vi "Multiple Connections - Server - TCP - 複製.vi"() -> ()   [LabVIEW 2011]
doc: "Demonstrates how to establish multiple connections and place them in a queue to be serviced. As connections are made, it sends the current date and time via TCP to all Client VIs that connect to it.\n\nThis VI has two parts -- a loop that listens for each client to connect, and a loop that sends the date and time to each connection in the queue.\n\n<B>Note:</B> Use this VI with Multiple Connections - Client 1.vi and Multiple Connections - Client 2.vi."
panel:
  out "# 2":i32
  in  "Port 2":u16=6342
  in  "stop":bool=TRUE
  out "# of Connections":i32
  in  "Port":u16=6341
  # "TCP Information"
  # "Instructions:\n1. Open the Multiple Connections - Client 1 and Client 2 VIs.\n2. Run this VI first.\n3. Run the Client VIs second and follow the instructions on their front panels.\n4. Stop This VI.  The Client VIs will stop on their own when they time out."
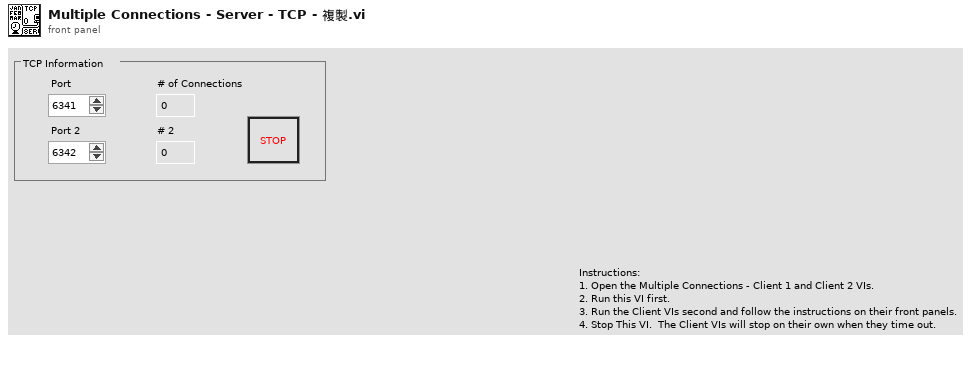
[diagram p1: front panel]
types:
  T1 = enum16{"Obtain", "Enqueue", "Dequeue", "Release"}
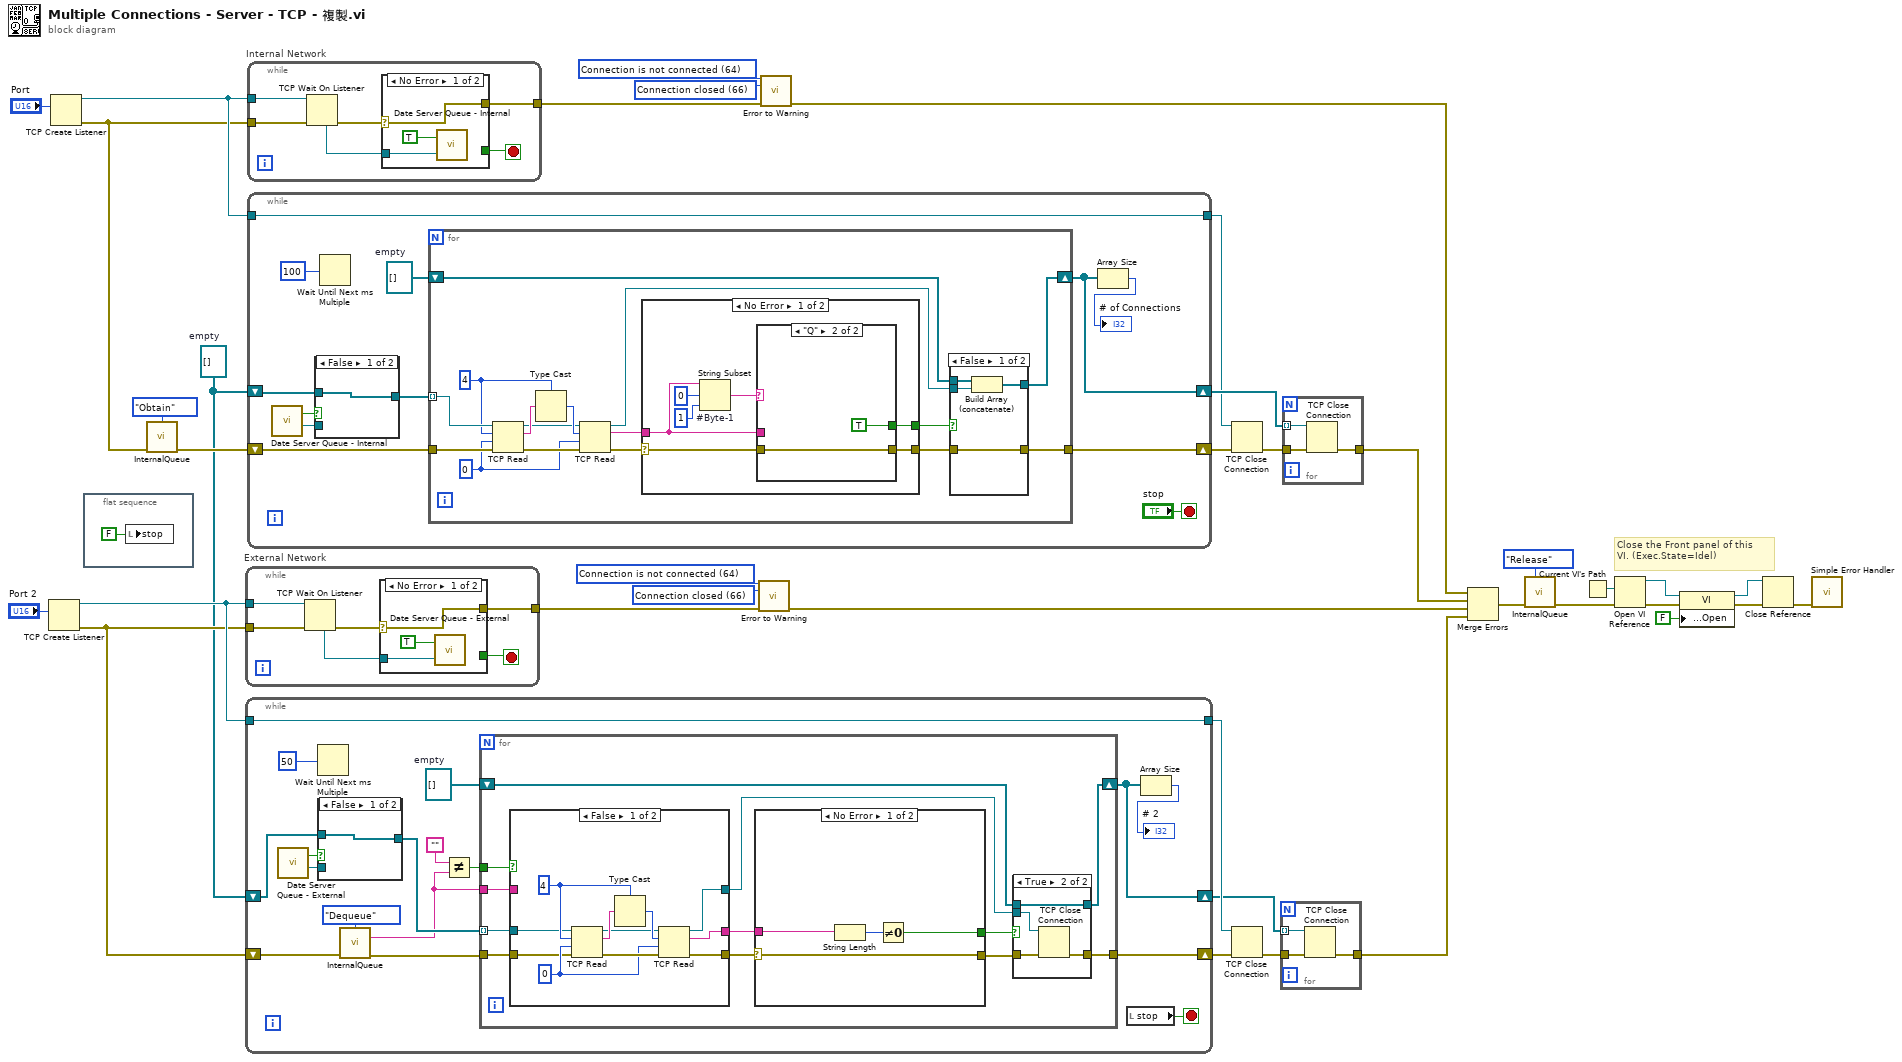
[diagram p0: block diagram]
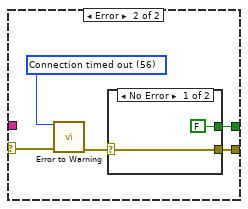
[diagram p2: hidden frame]
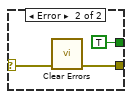
[diagram p3: hidden frame]
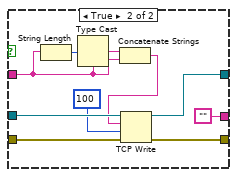
[diagram p4: hidden frame]
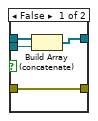
[diagram p5: hidden frame]
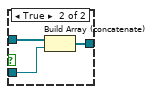
[diagram p6: hidden frame]
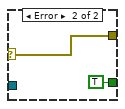
[diagram p7: hidden frame]
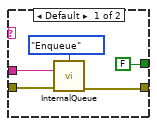
[diagram p8: hidden frame]
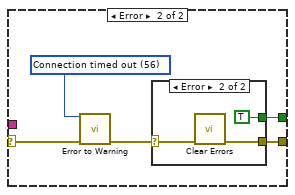
[diagram p9: hidden frame]
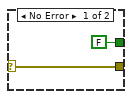
[diagram p10: hidden frame]
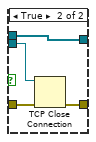
[diagram p11: hidden frame]
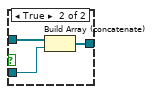
[diagram p12: hidden frame]
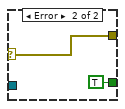
[diagram p13: hidden frame]
diagram:
  w20 = 66 items=["No Error", "Argument Error", "Memory Full", "Out of Zone", "End of File", "File Already Open", "Generic File IO Error", "File Not Found", "File Permission Error", "Disk Full", "Duplicate Path", "Too Many Files Open", "Not Enabled", "Resource File Not Found", "Cannot Add Resource", "Resource Not Found", "Image Not Found", "Image Memory Error", "Pen Does Not Exist", "Config Bad Type", "Config Token Not Found", "Config Parse Error", "Config Memory Error", "Bad External Code Format", "Bad External Code Offset", "External Code Not Present", "Null Window", "Destroy Window Mixup", "Null Menu", "Print Aborted", "Bad Print Record", "Print Driver Error", "Windows Error During Print", "Memory Error During Print", "Print Dialog Error", "Generic Print Error", "Invalid Device Refnum", "Device Not Found", "Device Parameter Error", "Device Unit Error", "Can't Open Device", "Device Call Aborted", "Generic Error", "Cancelled By User", "Object ID Too Low", "Object ID Too High", "Object Not In Heap", "Unknown Heap", "Bad DefProc ID", "DefProc Not In Table", "Message Out Of Range", "Null Method", "Unknown Message", "Manager Call Not Supported", "Bad address", "Connection In progress", "Connection timed out", "Connection is already in progress", "Network attribute not supported", "Network error", "Address in use", "System out of memory", "Connection aborted", "Connection refused", "Connection is not connected", "Connection is already connected", "Connection closed", "Initialize error (interapplication manager)", "Bad occurrence", "Wait on unbound occurrence handler", "Occurrence queue overflow", "Bad path", "Semaphore not signaled", "Unrecognized type (interapplication manager)"] ("2nd Error to Convert")
  w19 = 64 items=["No Error", "Argument Error", "Memory Full", "Out of Zone", "End of File", "File Already Open", "Generic File IO Error", "File Not Found", "File Permission Error", "Disk Full", "Duplicate Path", "Too Many Files Open", "Not Enabled", "Resource File Not Found", "Cannot Add Resource", "Resource Not Found", "Image Not Found", "Image Memory Error", "Pen Does Not Exist", "Config Bad Type", "Config Token Not Found", "Config Parse Error", "Config Memory Error", "Bad External Code Format", "Bad External Code Offset", "External Code Not Present", "Null Window", "Destroy Window Mixup", "Null Menu", "Print Aborted", "Bad Print Record", "Print Driver Error", "Windows Error During Print", "Memory Error During Print", "Print Dialog Error", "Generic Print Error", "Invalid Device Refnum", "Device Not Found", "Device Parameter Error", "Device Unit Error", "Can't Open Device", "Device Call Aborted", "Generic Error", "Cancelled By User", "Object ID Too Low", "Object ID Too High", "Object Not In Heap", "Unknown Heap", "Bad DefProc ID", "DefProc Not In Table", "Message Out Of Range", "Null Method", "Unknown Message", "Manager Call Not Supported", "Bad address", "Connection In progress", "Connection timed out", "Connection is already in progress", "Network attribute not supported", "Network error", "Address in use", "System out of memory", "Connection aborted", "Connection refused", "Connection is not connected", "Connection is already connected", "Connection closed", "Initialize error (interapplication manager)", "Bad occurrence", "Wait on unbound occurrence handler", "Occurrence queue overflow", "Bad path", "Semaphore not signaled", "Unrecognized type (interapplication manager)"] ("1st Error to Convert")
  w11 = refnum<k5>[] []  # empty
  w32 = 66 items=["No Error", "Argument Error", "Memory Full", "Out of Zone", "End of File", "File Already Open", "Generic File IO Error", "File Not Found", "File Permission Error", "Disk Full", "Duplicate Path", "Too Many Files Open", "Not Enabled", "Resource File Not Found", "Cannot Add Resource", "Resource Not Found", "Image Not Found", "Image Memory Error", "Pen Does Not Exist", "Config Bad Type", "Config Token Not Found", "Config Parse Error", "Config Memory Error", "Bad External Code Format", "Bad External Code Offset", "External Code Not Present", "Null Window", "Destroy Window Mixup", "Null Menu", "Print Aborted", "Bad Print Record", "Print Driver Error", "Windows Error During Print", "Memory Error During Print", "Print Dialog Error", "Generic Print Error", "Invalid Device Refnum", "Device Not Found", "Device Parameter Error", "Device Unit Error", "Can't Open Device", "Device Call Aborted", "Generic Error", "Cancelled By User", "Object ID Too Low", "Object ID Too High", "Object Not In Heap", "Unknown Heap", "Bad DefProc ID", "DefProc Not In Table", "Message Out Of Range", "Null Method", "Unknown Message", "Manager Call Not Supported", "Bad address", "Connection In progress", "Connection timed out", "Connection is already in progress", "Network attribute not supported", "Network error", "Address in use", "System out of memory", "Connection aborted", "Connection refused", "Connection is not connected", "Connection is already connected", "Connection closed", "Initialize error (interapplication manager)", "Bad occurrence", "Wait on unbound occurrence handler", "Occurrence queue overflow", "Bad path", "Semaphore not signaled", "Unrecognized type (interapplication manager)"] ("2nd Error to Convert")
  w33 = 64 items=["No Error", "Argument Error", "Memory Full", "Out of Zone", "End of File", "File Already Open", "Generic File IO Error", "File Not Found", "File Permission Error", "Disk Full", "Duplicate Path", "Too Many Files Open", "Not Enabled", "Resource File Not Found", "Cannot Add Resource", "Resource Not Found", "Image Not Found", "Image Memory Error", "Pen Does Not Exist", "Config Bad Type", "Config Token Not Found", "Config Parse Error", "Config Memory Error", "Bad External Code Format", "Bad External Code Offset", "External Code Not Present", "Null Window", "Destroy Window Mixup", "Null Menu", "Print Aborted", "Bad Print Record", "Print Driver Error", "Windows Error During Print", "Memory Error During Print", "Print Dialog Error", "Generic Print Error", "Invalid Device Refnum", "Device Not Found", "Device Parameter Error", "Device Unit Error", "Can't Open Device", "Device Call Aborted", "Generic Error", "Cancelled By User", "Object ID Too Low", "Object ID Too High", "Object Not In Heap", "Unknown Heap", "Bad DefProc ID", "DefProc Not In Table", "Message Out Of Range", "Null Method", "Unknown Message", "Manager Call Not Supported", "Bad address", "Connection In progress", "Connection timed out", "Connection is already in progress", "Network attribute not supported", "Network error", "Address in use", "System out of memory", "Connection aborted", "Connection refused", "Connection is not connected", "Connection is already connected", "Connection closed", "Initialize error (interapplication manager)", "Bad occurrence", "Wait on unbound occurrence handler", "Occurrence queue overflow", "Bad path", "Semaphore not signaled", "Unrecognized type (interapplication manager)"] ("1st Error to Convert")
  # "Close the Front panel of this\nVI. (Exec.State=Idel)"
  n1 = TCP Create Listener(10:"Port 2") -> (0:w12:errorcluster, 3:w17:refnum<k5>)  [unwired: 1 in, 4 out]
  n2 = TCP Create Listener(10:"Port") -> (0:w26:errorcluster, 3:w35:refnum<k5>)  [unwired: 1 in, 4 out]
  n3 = flat-sequence {
    frame #0 {
      n4 = local write "stop"(FALSE ("stop")) -> ()
    }
  }
  n5 = call "InternalQueue.vi"("Mode"=T1."Obtain", "error in (no error)"=w26) -> ("error out"=w28:errorcluster)  [unwired: 12 in, 1 out]
  n6 = while "External Network" {
    tunnel: w17 -> [w43]
    tunnel: w12 -> [w44]
    tunnel: [w39] -> w18
    stop <- w40 stop-if-true
    n7 = TCP Wait On Listener(8:w44, 11:w43) -> (0:w41:errorcluster, 4:w42:refnum<k5>)  [unwired: 5 out]
    n8 = case shown="No Error" w41 {
      selector: w41 -> [w45 w48]
      tunnel: w42 -> [w46 _]
      tunnel: [_ TRUE] -> w40
      tunnel: [w45 w48] -> w39
      frame No Error {
        n9 = call "Date Server Queue - External.vi"("new value"=w46, "set queue? (F: de-queue)"=TRUE) -> ()  [unwired: 2 out]
      }
      frame Error {
      }
    }
  }
  n10 = while {
    shift-left: w11 -> [w64]
    shift-right: [w61] -> w15
    tunnel: w17 -> [w59]
    tunnel: [w59] -> w16
    shift-right: [w58] -> w23
    shift-left: w12 -> [w56]
    stop <- w54 stop-if-true
    w62 = refnum<k5>[] []  # empty
    n11 = call "Date Server Queue - External.vi"() -> ("value"=w66:refnum<k5>, "valid?"=w65:bool)  [unwired: 2 in]
    n12 = Wait Until Next ms Multiple(millisecond multiple=u32 50) -> ()  [unwired: 1 out]
    n13 = case shown="False" w65 {
      tunnel: w66 -> [_ w125]
      tunnel: w64 -> [w122 w124]
      tunnel: [w122 w123] -> w63
      frame False {
      }
      frame True {
        n14 = Build Array (concatenate)(w124, w125) -> (w123:refnum<k5>[])
      }
    }
    n15 = call "InternalQueue.vi"("Mode"=T1."Dequeue", "error in (no error)"=w56) -> ("Queue Out"=w51:string, "error out"=w55:errorcluster)  [unwired: 12 in]
    n16 = Not Equal?(x="", y=w51) -> (x != y?=w50:bool)
    n17 = for {
      tunnel: w63 -> [w75] mode=indexing
      shift-right: [w76] -> w61
      shift-left: w62 -> [w78]
      tunnel: [w77] -> w58
      tunnel: w55 -> [w74]
      tunnel: w51 -> [w69]
      tunnel: w50 -> [w68]
      n18 = case shown="False" w68 {
        tunnel: w75 -> [w95 w109]
        tunnel: w74 -> [w97 w111]
        tunnel: [w96 w107] -> w73
        tunnel: w69 -> [_ w110]
        tunnel: [w93 w105] -> w67
        tunnel: [w94 ""] -> w70
        frame False {
          w98 = 0 ("timeout ms (25000)")
          w100 = 4
          n19 = TCP Read(connection ID=w95, bytes to read=w100, error in (no error)=w97, 9:w98) -> (connection ID out=w99:refnum<k5>, data out=w101:string, error out=w102:errorcluster)  [unwired: 1 out]
          n20 = Type Cast(type=w100, x=w101) -> (*(type *) &x=w103:i32)
          n21 = TCP Read(connection ID=w99, bytes to read=w103, error in (no error)=w102, 9:w98) -> (connection ID out=w93:refnum<k5>, data out=w94:string, error out=w96:errorcluster)  [unwired: 1 out]
        }
        frame True {
          n22 = String Length(string=w110) -> (length=w113:i32)
          n23 = Type Cast(type=w110, x=w113) -> (*(type *) &x=w112:string)
          n24 = Concatenate Strings(w112, w110) -> (w106:string)
          n25 = TCP Write(connection ID=w109, data in=w106, error in (no error)=w111, 9:100 ("timeout ms (25000)")) -> (connection ID out=w105:refnum<k5>, error out=w107:errorcluster)  [unwired: 1 out]
        }
      }
      n26 = case shown="No Error" w73 {
        selector: w73 -> [w82 w87]
        tunnel: [w82 w84] -> w71
        tunnel: [w79 w83] -> w72
        tunnel: w70 -> [w81 _]
        frame No Error {
          n27 = String Length(string=w81) -> (length=w80:i32)
          n28 = Not Equal To 0?(x=w80) -> (x != 0?=w79:bool)
        }
        frame Error {
          w86 = 56 items=["No Error", "Argument Error", "Memory Full", "Out of Zone", "End of File", "File Already Open", "Generic File IO Error", "File Not Found", "File Permission Error", "Disk Full", "Duplicate Path", "Too Many Files Open", "Not Enabled", "Resource File Not Found", "Cannot Add Resource", "Resource Not Found", "Image Not Found", "Image Memory Error", "Pen Does Not Exist", "Config Bad Type", "Config Token Not Found", "Config Parse Error", "Config Memory Error", "Bad External Code Format", "Bad External Code Offset", "External Code Not Present", "Null Window", "Destroy Window Mixup", "Null Menu", "Print Aborted", "Bad Print Record", "Print Driver Error", "Windows Error During Print", "Memory Error During Print", "Print Dialog Error", "Generic Print Error", "Invalid Device Refnum", "Device Not Found", "Device Parameter Error", "Device Unit Error", "Can't Open Device", "Device Call Aborted", "Generic Error", "Cancelled By User", "Object ID Too Low", "Object ID Too High", "Object Not In Heap", "Unknown Heap", "Bad DefProc ID", "DefProc Not In Table", "Message Out Of Range", "Null Method", "Unknown Message", "Manager Call Not Supported", "Bad address", "Connection In progress", "Connection timed out", "Connection is already in progress", "Network attribute not supported", "Network error", "Address in use", "System out of memory", "Connection aborted", "Connection refused", "Connection is not connected", "Connection is already connected", "Connection closed", "Initialize error (interapplication manager)", "Bad occurrence", "Wait on unbound occurrence handler", "Occurrence queue overflow", "Bad path", "Semaphore not signaled", "Unrecognized type (interapplication manager)"] ("1st Error to Convert")
          n29 = call <vilib>:"Error to Warning.vi"("1st Error to Convert"=w86, "error in"=w87) -> ("warning out"=w85:errorcluster)  [unwired: 13 in]
          n30 = case shown="No Error" w85 {
            selector: w85 -> [w89 w92]
            tunnel: [w89 w91] -> w84
            tunnel: [FALSE TRUE] -> w83
            frame No Error {
            }
            frame Error {
              n31 = call <vilib>:"Clear Errors.vi"("error in (no error)"=w92) -> ("error out"=w91:errorcluster)  [unwired: 6 in]
            }
          }
        }
      }
      n32 = case shown="True" w72 {
        tunnel: w78 -> [w117 w121]
        tunnel: w67 -> [w116 w120]
        tunnel: [w115 w121] -> w76
        tunnel: w71 -> [w114 w119]
        tunnel: [w114 w118] -> w77
        frame False {
          n33 = Build Array (concatenate)(w117, w116) -> (w115:refnum<k5>[])
        }
        frame True {
          n34 = TCP Close Connection(connection ID=w120, error in (no error)=w119) -> (error out=w118:errorcluster)  [unwired: 2 out]
        }
      }
    }
    n35 = local read "stop"() -> (w54:bool)
    n36 = Array Size(array=w61) -> (size(s)=→"# 2":i32)
  }
  n37 = while "Internal Network" {
    tunnel: w35 -> [w130]
    tunnel: w26 -> [w131]
    tunnel: [w126] -> w34
    stop <- w127 stop-if-true
    n38 = TCP Wait On Listener(8:w131, 11:w130) -> (0:w128:errorcluster, 4:w129:refnum<k5>)  [unwired: 5 out]
    n39 = case shown="No Error" w128 {
      selector: w128 -> [w132 w135]
      tunnel: w129 -> [w133 _]
      tunnel: [_ TRUE] -> w127
      tunnel: [w132 w135] -> w126
      frame No Error {
        n40 = call "Date Server Queue - Internal.vi"("new value"=w133, "set queue? (F: de-queue)"=TRUE) -> ()  [unwired: 2 out]
      }
      frame Error {
      }
    }
  }
  n41 = while {
    shift-left: w11 -> [w146]
    shift-right: [w143] -> w37
    tunnel: w35 -> [w141]
    tunnel: [w141] -> w36
    shift-right: [w138] -> w27
    shift-left: w28 -> [w139]
    stop <- "stop" stop-if-true
    w144 = refnum<k5>[] []  # empty
    n42 = call "Date Server Queue - Internal.vi"() -> ("value"=w148:refnum<k5>, "valid?"=w147:bool)  [unwired: 2 in]
    n43 = case shown="False" w147 {
      tunnel: w148 -> [_ w200]
      tunnel: w146 -> [w197 w199]
      tunnel: [w197 w198] -> w145
      frame False {
      }
      frame True {
        n44 = Build Array (concatenate)(w199, w200) -> (w198:refnum<k5>[])
      }
    }
    n45 = Wait Until Next ms Multiple(millisecond multiple=u32 100) -> ()  [unwired: 1 out]
    n46 = for {
      tunnel: w145 -> [w161] mode=indexing
      shift-right: [w163] -> w143
      shift-left: w144 -> [w164]
      tunnel: [w162] -> w138
      tunnel: w139 -> [w160]
      w149 = 0 ("timeout ms (25000)")
      w153 = 4
      n47 = TCP Read(connection ID=w161, bytes to read=w153, error in (no error)=w160, 9:w149) -> (connection ID out=w152:refnum<k5>, data out=w154:string, error out=w156:errorcluster)  [unwired: 1 out]
      n48 = Type Cast(type=w153, x=w154) -> (*(type *) &x=w157:i32)
      n49 = TCP Read(connection ID=w152, bytes to read=w157, error in (no error)=w156, 9:w149) -> (connection ID out=w150:refnum<k5>, data out=w151:string, error out=w155:errorcluster)  [unwired: 1 out]
      n50 = case shown="No Error" w155 {
        selector: w155 -> [w165 w182]
        tunnel: [w168 w181] -> w159
        tunnel: [w167 w179] -> w158
        tunnel: w151 -> [w166 _]
        frame No Error {
          n51 = String Subset "#Byte-1"(string=w166, offset (0)=0, length (rest)=1 ("length (rest)")) -> (substring=w169:string)
          n52 = case shown="\"Q\"" w169 {
            tunnel: w166 -> [w172 _]
            tunnel: w165 -> [w174 w178]
            tunnel: [w173 w178] -> w168
            tunnel: [FALSE TRUE] -> w167
            frame Default {
              n53 = call "InternalQueue.vi"("Mode"=T1."Enqueue", "Queue In"=w172, "error in (no error)"=w174) -> ("error out"=w173:errorcluster)  [unwired: 11 in, 1 out]
            }
            frame "Q" {
            }
          }
        }
        frame Error {
          w183 = 56 items=["No Error", "Argument Error", "Memory Full", "Out of Zone", "End of File", "File Already Open", "Generic File IO Error", "File Not Found", "File Permission Error", "Disk Full", "Duplicate Path", "Too Many Files Open", "Not Enabled", "Resource File Not Found", "Cannot Add Resource", "Resource Not Found", "Image Not Found", "Image Memory Error", "Pen Does Not Exist", "Config Bad Type", "Config Token Not Found", "Config Parse Error", "Config Memory Error", "Bad External Code Format", "Bad External Code Offset", "External Code Not Present", "Null Window", "Destroy Window Mixup", "Null Menu", "Print Aborted", "Bad Print Record", "Print Driver Error", "Windows Error During Print", "Memory Error During Print", "Print Dialog Error", "Generic Print Error", "Invalid Device Refnum", "Device Not Found", "Device Parameter Error", "Device Unit Error", "Can't Open Device", "Device Call Aborted", "Generic Error", "Cancelled By User", "Object ID Too Low", "Object ID Too High", "Object Not In Heap", "Unknown Heap", "Bad DefProc ID", "DefProc Not In Table", "Message Out Of Range", "Null Method", "Unknown Message", "Manager Call Not Supported", "Bad address", "Connection In progress", "Connection timed out", "Connection is already in progress", "Network attribute not supported", "Network error", "Address in use", "System out of memory", "Connection aborted", "Connection refused", "Connection is not connected", "Connection is already connected", "Connection closed", "Initialize error (interapplication manager)", "Bad occurrence", "Wait on unbound occurrence handler", "Occurrence queue overflow", "Bad path", "Semaphore not signaled", "Unrecognized type (interapplication manager)"] ("1st Error to Convert")
          n54 = call <vilib>:"Error to Warning.vi"("1st Error to Convert"=w183, "error in"=w182) -> ("warning out"=w180:errorcluster)  [unwired: 13 in]
          n55 = case shown="Error" w180 {
            selector: w180 -> [w185 w188]
            tunnel: [w185 w187] -> w181
            tunnel: [FALSE TRUE] -> w179
            frame No Error {
            }
            frame Error {
              n56 = call <vilib>:"Clear Errors.vi"("error in (no error)"=w188) -> ("error out"=w187:errorcluster)  [unwired: 6 in]
            }
          }
        }
      }
      n57 = case shown="False" w158 {
        tunnel: w164 -> [w192 w196]
        tunnel: w150 -> [w191 w195]
        tunnel: [w190 w196] -> w163
        tunnel: w159 -> [w189 w194]
        tunnel: [w189 w193] -> w162
        frame False {
          n58 = Build Array (concatenate)(w192, w191) -> (w190:refnum<k5>[])
        }
        frame True {
          n59 = TCP Close Connection(connection ID=w195, error in (no error)=w194) -> (error out=w193:errorcluster)  [unwired: 2 out]
        }
      }
    }
    n60 = Array Size(array=w143) -> (size(s)=→"# of Connections":i32)
  }
  n61 = call <vilib>:"Error to Warning.vi"("1st Error to Convert"=w19, "2nd Error to Convert"=w20, "error in"=w18) -> ("warning out"=w14:errorcluster)  [unwired: 2 in, 10 out]
  n62 = call <vilib>:"Error to Warning.vi"("1st Error to Convert"=w33, "2nd Error to Convert"=w32, "error in"=w34) -> ("warning out"=w29:errorcluster)  [unwired: 2 in, 10 out]
  n63 = TCP Close Connection(connection ID=w36, error in (no error)=w27) -> (error out=w30:errorcluster)  [unwired: 2 out]
  n64 = TCP Close Connection(connection ID=w16, error in (no error)=w23) -> (error out=w22:errorcluster)  [unwired: 2 out]
  n65 = for {
    tunnel: w15 -> [w203] mode=indexing
    tunnel: [w202] -> w13
    tunnel: w22 -> [w201]
    n66 = TCP Close Connection(connection ID=w203, error in (no error)=w201) -> (error out=w202:errorcluster)  [unwired: 2 out]
  }
  n67 = for {
    tunnel: w37 -> [w206] mode=indexing
    tunnel: [w205] -> w10
    tunnel: w30 -> [w204]
    n68 = TCP Close Connection(connection ID=w206, error in (no error)=w204) -> (error out=w205:errorcluster)  [unwired: 2 out]
  }
  n69 = Merge Errors(w29, w10, w14, w13) -> (w9:errorcluster)
  n70 = call "InternalQueue.vi"("Mode"=T1."Release", "error in (no error)"=w9) -> ("error out"=w1:errorcluster)  [unwired: 12 in, 1 out]
  n71 = Current VI's Path() -> (path=w8:path)
  n72 = Open VI Reference(vi path=w8, error in (no error)=w1) -> (vi reference=w3:refnum<vi>, error out=w7:errorcluster)  [unwired: 4 in]
  n73 = property class="VI"(reference=w3, error in=w7, "Front Panel Window:Open"=FALSE) -> (reference out=w6:refnum<vi>, error out=w4:errorcluster)
  n74 = Close Reference(reference=w6, error in (no error)=w4) -> (error out=w2:errorcluster)
  n75 = call <vilib>:"Simple Error Handler.vi"("error in (no error)"=w2) -> ()  [unwired: 1 in, 8 out]
